vi "Init.vi"(10 "Secret":string, 11 "ID":string) -> (3 "Client out":refnum<class "Client.lvclass">)   [LabVIEW 2020, in "OAuth2.lvlib" / "Client.lvclass"]
doc: "Initializes the client credentials that identify the application requesting authorization. These values are obtained by registering with the authorization provider."
uses:
  Client.lvclass
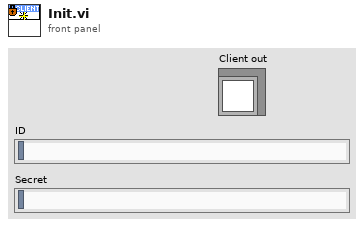
[diagram p1: front panel]
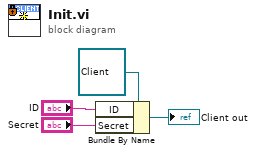
[diagram p0: block diagram]
diagram:
  n1 = Bundle By Name(cluster=refnum<class "Client.lvclass"> refnum ("Client out"), "ID"="ID", "Secret"="Secret") -> (→"Client out":refnum<class "Client.lvclass">)
